vi "Ctrl_Loop.vi"() -> ()   [LabVIEW 2018]
doc: "Runs the control loop at a deterministic loop rate. Implements discrete time PID controller using discrete-time transfer functions for the lead controller and custom-built integrator for the lag controller.\n\nAnalog Input/Output -\nC/AI0 : plant measurement\nC/AI1 : reference input\nC/AO0 : control effort out\nC/AO1 : error signal out\n\nController Optimized for speed\n- Probe signals using oscilloscope\n- Loop bode plot meas. using oscilloscope"
uses:
  <vilib>/Platform/TimedLoop/XDataNode/timing_clust.ctl
  <vilib>/Platform/TimedLoop/XDataNode/nitl_modes.ctl
  <vilib>/Platform/TimedLoop/XDataNode/wakeup.ctl
  <vilib>/myRIO/Instrument Drivers/Onboard IO/AO/typedefs/AO Reference.ctl
  <vilib>/myRIO/Common/Instrument Driver Framework/Utilities/typedefs/myRIO Generic Hardware Reference.ctl
  <vilib>/myRIO/Common/Instrument Driver Framework/Utilities/typedefs/Hardware Version Enum.ctl
  <vilib>/myRIO/Common/Instrument Driver Framework/Utilities/typedefs/myRIO v1.0 Reference.ctl
  <vilib>/myRIO/Common/Instrument Driver Framework/Utilities/typedefs/Generic FPGA Reference.ctl
  <vilib>/myRIO/Common/Instrument Driver Framework/myRIO v1.0/AO/typedefs/AO Channels List.ctl
  <vilib>/myRIO/Common/Instrument Driver Framework/myRIO v1.0/AO/typedefs/AO Channels Enum.ctl
  <vilib>/myRIO/Common/Instrument Driver Framework/Utilities/typedefs/Analog Scaling Constants List.ctl
  <vilib>/myRIO/Common/Instrument Driver Framework/Utilities/typedefs/Analog Scaling Constants.ctl
  <vilib>/userdefined/High Color/nirio_resource_hc.ctl
  <vilib>/myRIO/Instrument Drivers/Onboard IO/AI/typedefs/AI Reference.ctl
  <vilib>/myRIO/Common/Instrument Driver Framework/myRIO v1.0/AI/typedefs/AI Channels List.ctl
  <vilib>/myRIO/Common/Instrument Driver Framework/myRIO v1.0/AI/typedefs/AI Channels Enum.ctl
  Components/Controllers/TF_diff_mode.ctl
  <vilib>/myRIO/Common/Instrument Driver Framework/myRIO v1.0/AO/vis/myRIO v1.1 Open AO.vi
  <vilib>/myRIO/Common/Instrument Driver Framework/myRIO v1.0/AI/vis/myRIO v1.1 Open AI.vi
  <vilib>/Simulation/DiscreteLinear/Implementation/NILVSim Discrete Transfer Function Direct.llb/SIM Discrete Transfer Function Diagram (SISO).vi
  <vilib>/myRIO/Common/Instrument Driver Framework/Utilities/vis/Validate Channels.vi
  <vilib>/myRIO/Common/Instrument Driver Framework/myRIO v1.0/AO/vis/myRIO v1.0 Reserve AO.vi
  <vilib>/myRIO/Common/Instrument Driver Framework/myRIO v1.0/AI/vis/myRIO v1.0 Reserve AI.vi
  <vilib>/Simulation/ContinuousLinear/Implementation/Shared/SIM Transfer Function Support.llb/SIM TransferFunction Normalize to Buffer.vi
  <vilib>/Simulation/DiscreteLinear/Implementation/Shared/SIM Init Discrete States.vi
  <vilib>/Simulation/DiscreteLinear/Implementation/NILVSim Discrete Transfer Function Direct.llb/SIM Transfer Function Direct core (SISO).vi
  <vilib>/myRIO/Common/Instrument Driver Framework/myRIO v1.0/AO/vis/myRIO v1.0 Close AO.vi
  <vilib>/myRIO/Common/Instrument Driver Framework/myRIO v1.0/AI/vis/myRIO v1.0 Close AI.vi
  <vilib>/myRIO/Common/Instrument Driver Framework/myRIO v1.0/AO/vis/myRIO v1.0 Build MUX Configuration AO.vi
  <vilib>/myRIO/Common/Instrument Driver Framework/myRIO v1.0/Resource Manager/vis/myRIO v1.0 Reserve Channel List.vi
  <vilib>/myRIO/Common/Instrument Driver Framework/myRIO v1.0/AI/vis/myRIO v1.0 Build MUX Configuration AI.vi
  <vilib>/Simulation/ContinuousLinear/Implementation/Shared/SIM Transfer Function Support.llb/SIM TransferFunction Normalize.vi
  <vilib>/myRIO/Common/Instrument Driver Framework/myRIO v1.0/AO/vis/myRIO v1.0 Unreserve AO.vi
  <vilib>/myRIO/Common/Instrument Driver Framework/myRIO v1.0/AI/vis/myRIO v1.0 Unreserve AI.vi
  <vilib>/myRIO/Common/Instrument Driver Framework/myRIO v1.0/Resource Manager/vis/myRIO v1.0 Reserve Channel.vi
  <vilib>/myRIO/Common/Instrument Driver Framework/myRIO v1.0/Resource Manager/vis/myRIO v1.0 Unreserve Channel.vi
  <vilib>/Simulation/Implementation/Shared/SIM Polynomials.llb/SIM Remove Zero Coefficients (DBL).vi
  <vilib>/myRIO/Common/Instrument Driver Framework/myRIO v1.0/Resource Manager/vis/myRIO v1.0 Unreserve Channel List.vi
  <vilib>/myRIO/Common/Instrument Driver Framework/myRIO v1.0/Resource Manager/vis/myRIO v1.0 Build Mutex Name.vi
  <vilib>/Utility/VariantDataType/GetNumericInfo.vi
  <vilib>/Utility/error.llb/Error Cluster From Error Code.vi
  <vilib>/myRIO/Common/Instrument Driver Framework/myRIO v1.0/myRIO v1.1 Open.vi
  <vilib>/myRIO/Common/Instrument Driver Framework/myRIO v1.0/AI/vis/myRIO v1.0 Get Scaling Constants AI.vi
  <vilib>/myRIO/Common/Instrument Driver Framework/Utilities/vis/IO Manager.vi
  <vilib>/myRIO/Common/Instrument Driver Framework/Utilities/vis/Configuration Manager.vi
  <vilib>/myRIO/Common/Instrument Driver Framework/myRIO v1.0/myRIO v1.0 Close.vi
  <vilib>/myRIO/Common/Instrument Driver Framework/myRIO v1.0/AO/vis/myRIO v1.0 Get Scaling Constants AO.vi
  <vilib>/myRIO/Common/Instrument Driver Framework/myRIO v1.0/AI/vis/myRIO v1.0 Read AI.vi
  <vilib>/Simulation/Implementation/Shared/SIM Polynomials.llb/SIM Divide Polynomials (DBL).vi
  <vilib>/Simulation/Implementation/Shared/SIM BuildSimErr.vi
  <vilib>/myRIO/Common/Instrument Driver Framework/myRIO v1.0/AO/vis/myRIO v1.0 Write AO.vi
  <vilib>/platform/TimedLoop/XDataNode/XDataNode.xnode
  <vilib>/myRIO/Instrument Drivers/Onboard IO/AI/vis/myRIO AI Open.xnode
  <vilib>/myRIO/Instrument Drivers/Onboard IO/AO/vis/myRIO AO Open.xnode
  <vilib>/Simulation/Implementation/XNodeFramework/SimXNode/SimX.xnode
  <vilib>/Platform/TimedLoop/XDataNode/XDNodeRunTimeDep.lvlib
  <vilib>/myRIO/Instrument Drivers/Onboard IO/AI/AI.lvlib
  <vilib>/myRIO/Instrument Drivers/Onboard IO/AO/AO.lvlib
  components/Controllers/DiscreteControllers.lvlib
  Components/Boolean functions/Boolean Functions.lvlib
panel:
  out "Loop rate [Hz]":dbl format="%#.0f"
  in  "Controller On?":bool
  in  "Kp":dbl=1.0
  out "Sample Time [s]":dbl format="%#_8f"
  in  "System Stop Button":bool
  out "# of loops late":i16
  # "Controller Optimized for speed\n- Probe signals using oscilloscope\n- Loop bode plot meas. using \n   oscilloscope\n- See context help (Ctrl+H), hover\n   over icon for more information."
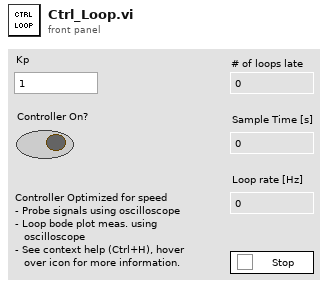
[diagram p1: front panel]
types:
  T1 = typedef "XDNodeRunTimeDep.lvlib/timing_clust.ctl" = cluster{"Expected End [f-1]":u64, "Actual End [f-1]":u64, "Finished Late? [f-1]":bool, "Expected End [i-1]":u64, "Actual End [i-1]":u64, "Finished Late? [i-1]":bool, "Expected Start [i]":u64, "Actual Start [i]":u64, "Expected Start [f]":u64, "Actual Start [f]":u64, "Source Name":string, "Structure Name":string, "Period":i64, "Deadline":i64, "Offset":i64, "Start":i64, "Priority":i32, "Timeout":i32, "Mode":T2, "Wakeup Reason":T3, "Error":errorcluster, "Source Type":string, "Secondary Source Type":string, "Global End Time":u64, "Global Start Time":u64, "Frame Duration":u64, "Iteration Duration":u64, "Assigned CPU":i32, "I/O Scan Engine Mode":u32}
  T2 = typedef "XDNodeRunTimeDep.lvlib/nitl_modes.ctl" = enum32{"No Change", "Process missed periods, maintain original phase", "Discard missed periods, maintain original phase", "Process missed periods, ignore original phase", "Discard missed periods, ignore original phase"}
  T3 = typedef "XDNodeRunTimeDep.lvlib/wakeup.ctl" = enum32{"Normal", "Aborted", "Asynchronous wakeup", "Timing source error", "Timed loop error", "Timeout"}
  T4 = typedef "AI.lvlib/AI Reference.ctl" = cluster{"myRIO Reference":T5, "AI Channels List":T9, "AI Scaling Constants List":T11}
  T5 = typedef "myRIO Generic Hardware Reference.ctl" = cluster{"myRIO Model":T6, "myRIO Hardware Reference":T7}
  T6 = typedef "Hardware Version Enum.ctl" = enum16{"Unknown", "myRIO-1900", "myRIO-1950", "roboRIO", "NI ELVIS RIO CM", "ELVIS III"}
  T7 = typedef "myRIO v1.0 Reference.ctl" = cluster{"Generic FPGA Reference":T8, "Allow multiple opens":bool}
  T8 = typedef "Generic FPGA Reference.ctl" = refnum<k20>
  T9 = typedef "AI Channels List.ctl" = T10[]
  T10 = typedef "AI Channels Enum.ctl" = enum16{"Not Connected", "AudioIn/Left", "AudioIn/Right", "C/AI0", "C/AI1", "A/AI0", "A/AI1", "A/AI2", "A/AI3", "A/AI4", "A/AI5", "A/AI6", "A/AI7", "B/AI0", "B/AI1", "B/AI2", "B/AI3", "B/AI4", "B/AI5", "B/AI6", "B/AI7", "AI/AI0", "AI/AI1", "AI/AI2", "AI/AI3", "A/AI0 (DIFF)", "A/AI1 (DIFF)", "A/AI2 (DIFF)", "A/AI3 (DIFF)", "B/AI0 (DIFF)", "B/AI1 (DIFF)", "B/AI2 (DIFF)", "B/AI3 (DIFF)"}
  T11 = typedef "Analog Scaling Constants List.ctl" = T12[]
  T12 = typedef "Analog Scaling Constants.ctl" = cluster{"LSB Weight (Volts)":dbl, "Offset (Volts)":dbl, "Signed?":bool}
  T13 = typedef "AO.lvlib/AO Reference.ctl" = cluster{"myRIO Reference":T5, "AO Channel List":T14, "AO Scaling Constant List":T11}
  T14 = typedef "AO Channels List.ctl" = T15[]
  T15 = typedef "AO Channels Enum.ctl" = enum16{"Not Connected", "AudioOut/Left", "AudioOut/Right", "C/AO0", "C/AO1", "A/AO0", "A/AO1", "B/AO0", "B/AO1"}
  T16 = typedef "DiscreteControllers.lvlib/TF_diff_mode.ctl" = enum16{"Forward Euler", "Backward Euler", "Tustin (Bilinear)"}
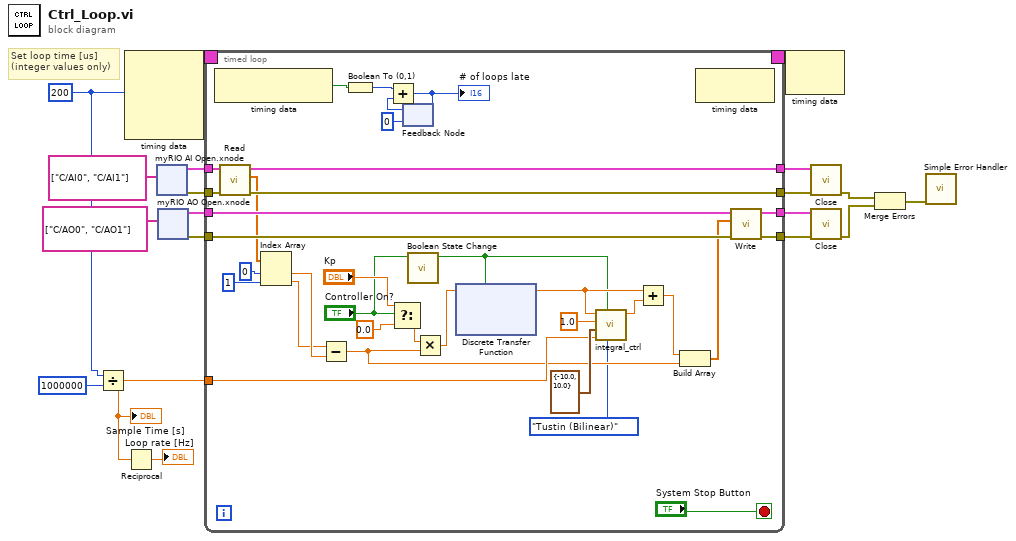
[diagram p0: block diagram]
diagram:
  w3 = i64 200 ("Period")
  # "Set loop time [us]\n(integer values only)"
  n1 = Divide(x=w3, y=i64 1000000) -> (x/y=w2:dbl)
  "Sample Time [s]" <- w2
  n2 = node-c288(w3) -> (w19:T1)  [unwired: 3 in]
  n3 = Reciprocal(x=w2) -> (1/x=→"Loop rate [Hz]":dbl)
  n4 = xnode "myRIO AI Open.xnode"("Channel Names"=tag[] ["C/AI0", "C/AI1"]) -> ("error out"=w15:errorcluster, "AI Ref Out"=w16:T4)  [unwired: 2 in]
  n5 = xnode "myRIO AO Open.xnode"("Channel Names"=tag[] ["C/AO0", "C/AO1"]) -> ("error out"=w9:errorcluster, "AO Ref Out"=w11:T13)  [unwired: 2 in]
  n6 = timed-loop {
    timing: w19 -> [_]
    timing-out: [_] -> w18
    tunnel: w16 -> [w53]
    tunnel: w15 -> [w52]
    tunnel: [w51] -> w14
    tunnel: [w49] -> w13
    tunnel: w11 -> [w48]
    tunnel: [w47] -> w10
    tunnel: w9 -> [w46]
    tunnel: [w45] -> w8
    tunnel: w2 -> [w30]
    stop <- "System Stop Button" stop-if-true
    n7 = node-c288() -> (w42:bool)  [unwired: 1 in]
    n8 = call <vilib>:"Read.vi"("error in (no error)"=w52, "AI Ref In"=w53) -> ("error out"=w49:errorcluster, "Values"=w44:dbl[], "AI Ref Out"=w51:T4)  [unwired: 7 in]
    n9 = Index Array(array=w44, index #1=0 ("index"), index #2=1 ("index")) -> (element #1=w35:dbl, element #2=w34:dbl)
    n10 = Subtract(x=w34, y=w35) -> (x-y=w29:dbl)
    n11 = Boolean To (0,1)(Boolean=w42) -> (0, 1=w41:i16)
    n12 = Select(t="Kp", s="Controller On?", f=0.0) -> (s? t:f=w28:dbl)
    n13 = feedback #1(i16 0) -> (w39:i16)
    n14 = Add(x=w41, y=w39) -> (x+y=w40:i16)
    "# of loops late" <- w40
    n15 = feedback-in #1(w40) -> ()
    n16 = call "Boolean State Change.vi"("Bool In"="Controller On?") -> ("State Change?"=w20:bool)  [unwired: 10 in]
    n17 = Multiply(x=w28, y=w29) -> (x*y=w27:dbl)
    n18 = xnode ("Discrete Transfer Function")("input u(k)"=w27, "initialize"=w20) -> ("output y(k)"=w25:dbl)  [unwired: 1 in, 1 out]
    n19 = call "integral_ctrl.vi"("Mode"=TF_diff_mode."Tustin (Bilinear)", "Initialize?"=w20, "Sampling \nTime"=w30, "Anti-windup limits"=cluster{"Lower limit":dbl, "Upper limit":dbl} {"Lower limit"=-10.0, "Upper limit"=10.0}, "Ki"=1.0, "Input"=w25) -> ("Output"=w24:dbl)  [unwired: 4 in, 1 out]
    n20 = Add(x=w25, y=w24) -> (x+y=w23:dbl)
    n21 = Build Array(w23, w29) -> (w43:dbl[])
    n22 = node-c288() -> ()  [unwired: 1 in, 1 out]
    n23 = call <vilib>:"Write.vi"("error in (no error)"=w46, "Values"=w43, "AO Ref In"=w48) -> ("error out"=w45:errorcluster, "AO Ref Out"=w47:T13)  [unwired: 6 in]
  }
  n24 = node-c288(w18) -> ()  [unwired: 1 out]
  n25 = call <vilib>:"Close.vi"("error in (no error)"=w13, "AI Ref In"=w14) -> ("error out"=w6:errorcluster)  [unwired: 9 in]
  n26 = call <vilib>:"Close.vi"("error in (no error)"=w8, "AO Ref In"=w10) -> ("error out"=w5:errorcluster)  [unwired: 9 in]
  n27 = Merge Errors(w6, w5) -> (w4:errorcluster)
  n28 = call <vilib>:"Simple Error Handler.vi"("error in (no error)"=w4) -> ()  [unwired: 4 in, 5 out]
